vi "Write Meta Data (Serial Clst).vi"(6 "options":T3={"ignore timeout error"=TRUE, "timeout ms (1000)"=1000}, 7 "meta data":T2[](array[typedef]), 8 "error in":errorcluster, 11 "connection info in":T1) -> (0 "error out":errorcluster, 3 "connection info out":T1)   [LabVIEW 2010, in "NI STM.lvlib"]
doc: "Use this VI to transmit the meta data cluster to a remote computer. Sending the meta data to another computer helps maintainability since the data resides only on one side and it is shared to other computers at run time."
uses:
  NI STM.lvlib
  Serial Connection Info.ctl
  SubVIs/MetaDataElement.ctl
  Serial Write Options.ctl
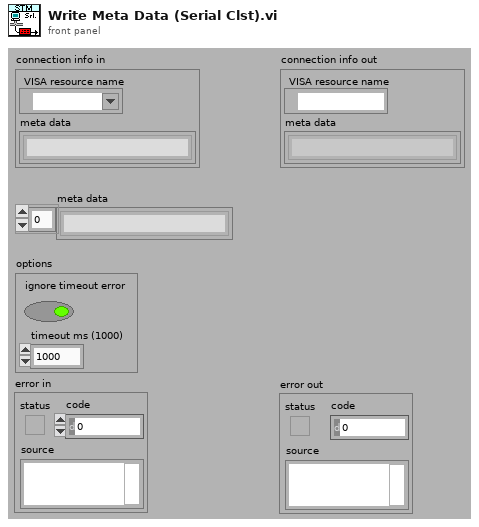
[diagram p1: front panel]
types:
  T1 = typedef "NI STM.lvlib/Serial Connection Info.ctl" = cluster{"VISA resource name":refnum<visa-resource-name>, "meta data":T2[]}
  T2 = typedef "NI STM.lvlib/MetaDataElement.ctl" = string
  T3 = typedef "NI STM.lvlib/Serial Write Options.ctl" = cluster{"ignore timeout error":bool, "timeout ms (1000)":u32}
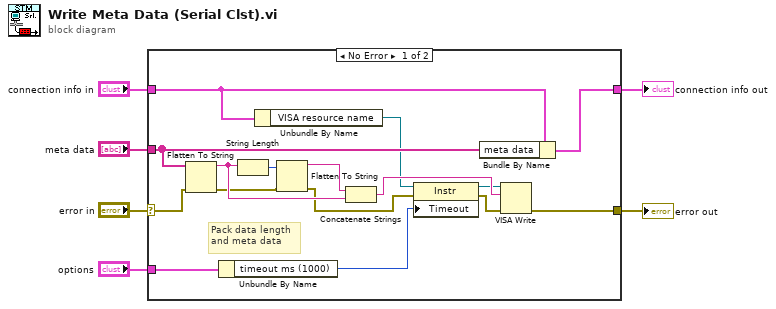
[diagram p0: block diagram]
diagram:
  n1 = case shown="No Error" "error in" {
    selector: "error in" -> [w14 w24]
    tunnel: [w16 w23] -> w6
    tunnel: "connection info in" -> [w12 w23]
    tunnel: "meta data" -> [w15 _]
    tunnel: [w22 w24] -> w4
    tunnel: "options" -> [w17 _]
    frame No Error {
      # "Pack data length\nand meta data"
      n2 = Flatten To String(anything=w15, error in (no error)=w14) -> (data string=w18:string, error out=w13:errorcluster)  [unwired: 3 out]
      n3 = Unbundle By Name(w17) -> ("timeout ms (1000)"=w9:u32)
      n4 = String Length(string=w18) -> (length=w21:i32)
      n5 = Unbundle By Name(w12) -> ("VISA resource name"=w11:refnum<visa-resource-name>)
      n6 = Flatten To String(anything=w21, error in (no error)=w13) -> (data string=w20:string, error out=w8:errorcluster)  [unwired: 3 out]
      n7 = Concatenate Strings(w20, w18) -> (w19:string)
      n8 = property class="Instr"(reference=w11, error in=w8, "Timeout"=w9) -> (reference out=w10:refnum<visa-resource-name>, error out=w7:errorcluster)
      n9 = Bundle By Name(cluster=w12, "meta data"=w15) -> (w16:T1)
      n10 = VISA Write(VISA resource name=w10, write buffer=w19, error in (no error)=w7) -> (error out=w22:errorcluster)  [unwired: 2 out]
    }
    frame Error {
    }
  }
  "connection info out" <- w6
  "error out" <- w4
